vi "Scan SFC.vi"() -> (1 "Ok?":bool, 3 "SFC Out":string)   [LabVIEW 2024]
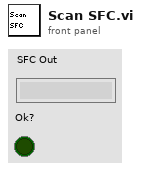
[diagram p1: front panel]
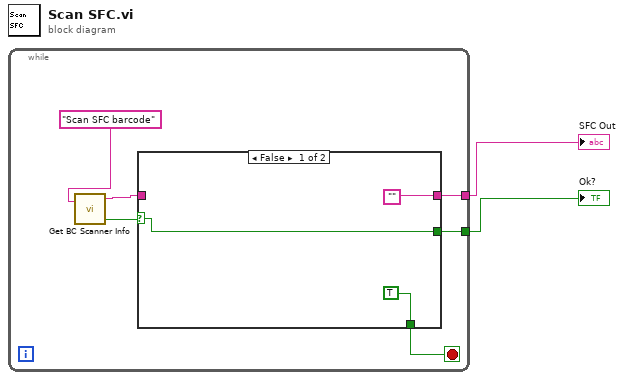
[diagram p0: block diagram]
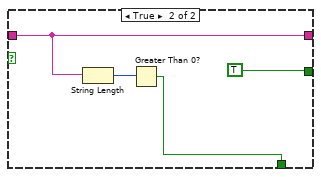
[diagram p2: hidden frame]
diagram:
  n1 = while {
    tunnel: [w5] -> w2
    tunnel: [w4] -> w1
    stop <- w3 stop-if-true
    n2 = call "Get BC Scanner Info.vi"("Prompt"="Scan SFC barcode") -> ("Info Out"=w7:string, "OK"=w6:bool)  [unwired: 2 in]
    n3 = case shown="False" w6 {
      selector: w6 -> [w11 _]
      tunnel: w7 -> [_ w14]
      tunnel: ["" w14] -> w5
      tunnel: [w11 TRUE] -> w4
      tunnel: [TRUE w12] -> w3
      frame False {
      }
      frame True {
        n4 = String Length(string=w14) -> (length=w13:i32)
        n5 = Greater Than 0?(x=w13) -> (x > 0?=w12:bool)
      }
    }
  }
  "SFC Out" <- w2
  "Ok?" <- w1
